vi "setFreq.vi"(3 "error in":errorcluster, 5 "Frequenz in Hz":dbl=200.0 format="%.2f", 6 "address string":string="19") -> (0 "error out":errorcluster)   [LabVIEW 2010]
panel:
  in  "mode (0)":i16
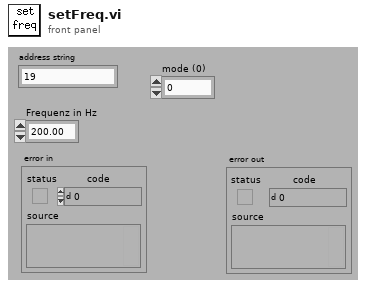
[diagram p1: front panel]
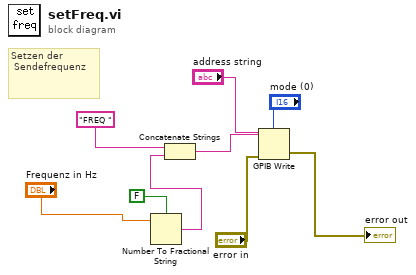
[diagram p0: block diagram]
diagram:
  # "Setzen der \n Sendefrequenz"
  n1 = Number To Fractional String(use system decimal point (T)=FALSE, number="Frequenz in Hz") -> (F-format string=w7:string)  [unwired: 2 in]
  n2 = Concatenate Strings("FREQ ", w7) -> (w8:string)
  n3 = GPIB Write(0:"address string", 1:w8, 2:"mode (0)", 3:"error in") -> (6:→"error out":errorcluster)  [unwired: 1 in, 1 out]
